vi "test Passes If Strings Are Equal.vi"(8 "error in (no error)":errorcluster, 11 "TestCase in":refnum<class "String Equality Test Case.lvclass">) -> (0 "error out":errorcluster, 3 "TestCase out":refnum<class "String Equality Test Case.lvclass">)   [LabVIEW 2015, in "String Equality Test Case.lvclass"]
uses:
  String Equality Test Case.lvclass
  <vilib>/addons/_JKI Toolkits/VI Tester/TestCase.llb/TestCase.lvclass
  VITAC.lvlib
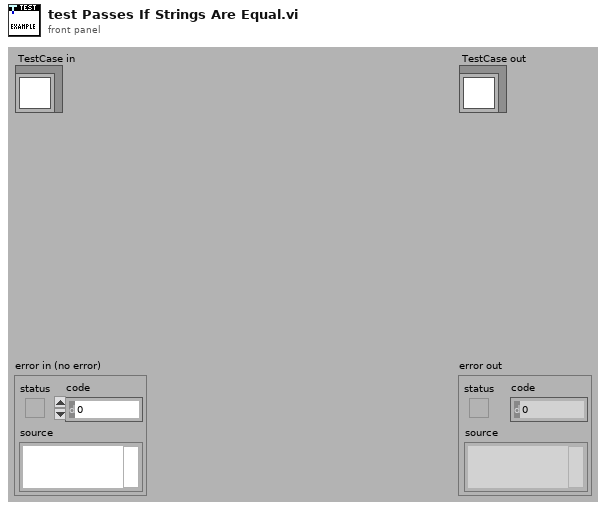
[diagram p1: front panel]
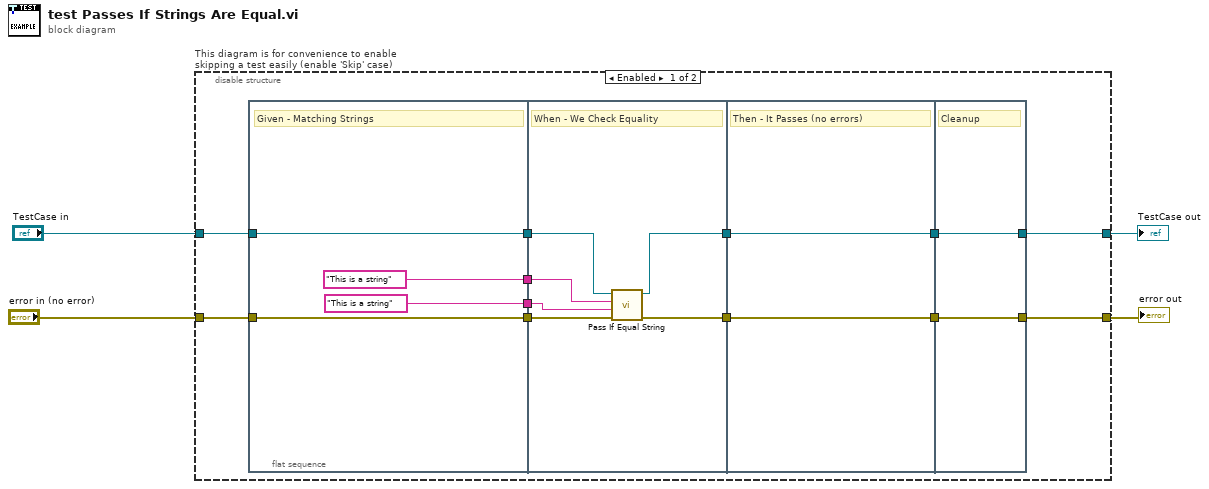
[diagram p0: block diagram]
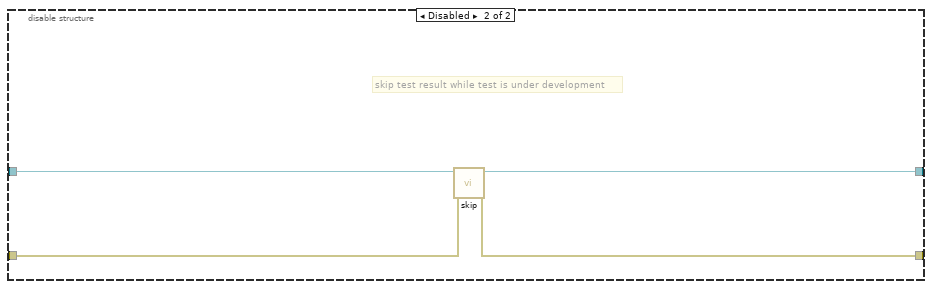
[diagram p2: hidden frame]
diagram:
  n1 = disable-structure "This diagram is for convenience to enable skipping a test easily (enable 'Skip' case)" shown="Enabled" {
    disable-tunnel: "TestCase in" -> [w16 w34]
    disable-tunnel: [w15 w32] -> w1
    disable-tunnel: [w14 w33] -> w3
    disable-tunnel: "error in (no error)" -> [w13 w31]
    frame Enabled {
      n2 = flat-sequence {
        tunnel: w13 -> [w19]
        tunnel: w16 -> [w20]
        tunnel: [w20] -> w8
        tunnel: [w19] -> w7
        tunnel: ["This is a string" ("expected")] -> w6
        tunnel: ["This is a string" ("expected")] -> w5
        tunnel: [w23] -> w10
        tunnel: [w25] -> w9
        tunnel: w8 -> [w24]
        tunnel: w7 -> [w26]
        tunnel: w6 -> [w22]
        tunnel: w5 -> [w21]
        tunnel: [w28] -> w12
        tunnel: [w27] -> w11
        tunnel: w10 -> [w28]
        tunnel: w9 -> [w27]
        tunnel: [w29] -> w14
        tunnel: [w30] -> w15
        tunnel: w12 -> [w30]
        tunnel: w11 -> [w29]
        frame #0 {
          # "Given - Matching Strings"
        }
        frame #1 {
          # "When - We Check Equality"
          n3 = call "Pass If Equal String.vi"("error in (no error)"=w26, "actual"=w21, "expected"=w22, "TestCase in"=w24) -> ("error out"=w25:errorcluster, "TestCase out"=w23:refnum<class "String Equality Test Case.lvclass">)  [unwired: 6 in]
        }
        frame #2 {
          # "Then - It Passes (no errors)"
        }
        frame #3 {
          # "Cleanup"
        }
      }
    }
    frame Disabled {
      # "skip test result while test is under development"
      n4 = call <vilib>:"skip.vi"("error in (no error)"=w31, "TestCase in"=w34) -> ("error out"=w33:errorcluster, "TestCase out"=w32:refnum<class "String Equality Test Case.lvclass">)  [unwired: 8 in]
    }
  }
  "error out" <- w3
  "TestCase out" <- w1
